vi "gui for machine parameters.vi"() -> ()   [LabVIEW 2022 SP3]
uses:
  <vilib>/picture/picture.llb/Draw True-Color Pixmap.vi
  horizontal slide control.ctl
  <vilib>/picture/picture.llb/imagedata.ctl
panel:
  in  "stop 3":bool
  in  "dimension size":i32
  in  "Tank 3":dbl(slide) scale=0.0..100.0
  in  "Tank 2":dbl(slide) scale=0.0..100.0
  in  "Table 3":string[][](table)
  in  "?":bool
  in  "?":bool
  in  "?":bool
  in  "?":bool
  in  "?":bool
  in  "?":bool
  in  "?":bool
  in  "?":bool
  out "image data 2":T1
  in  "path to PNG file 2":path=path "C:/Dhanush/Dhanush/Vehicle articulated (1).PNG"
  in  "Rotation Angle (degree) 2":dbl(knob) scale=-180.0..180.0
  in  "Scale 2":dbl(slide)=1.0 scale=0.1..10.0
  in  "stop 2":bool
  out "?":picture
  out "image data":T1
  in  "path to PNG file":path=path "C:/Dhanush/Dhanush/Vehicle articulated (1).PNG"
  in  "Rotation Angle (degree)":dbl(knob) scale=-180.0..180.0
  in  "Scale":dbl(slide)=1.0 scale=0.1..10.0
  in  "stop":bool
  out "?":picture
  out "?":T2 scale=0.0..100.0
  in  "Table 2":string[][](table)
  # "No of Cycles"
  # "Holding Time"
  # "Y axis Angle"
  # "Pressure"
  # "Automatic Mode Parameter Settings"
  # "Y axis"
  # "X axis"
  # "Cycle"
  # "Settings"
  # "%"
  # "Overall Progress Bar"
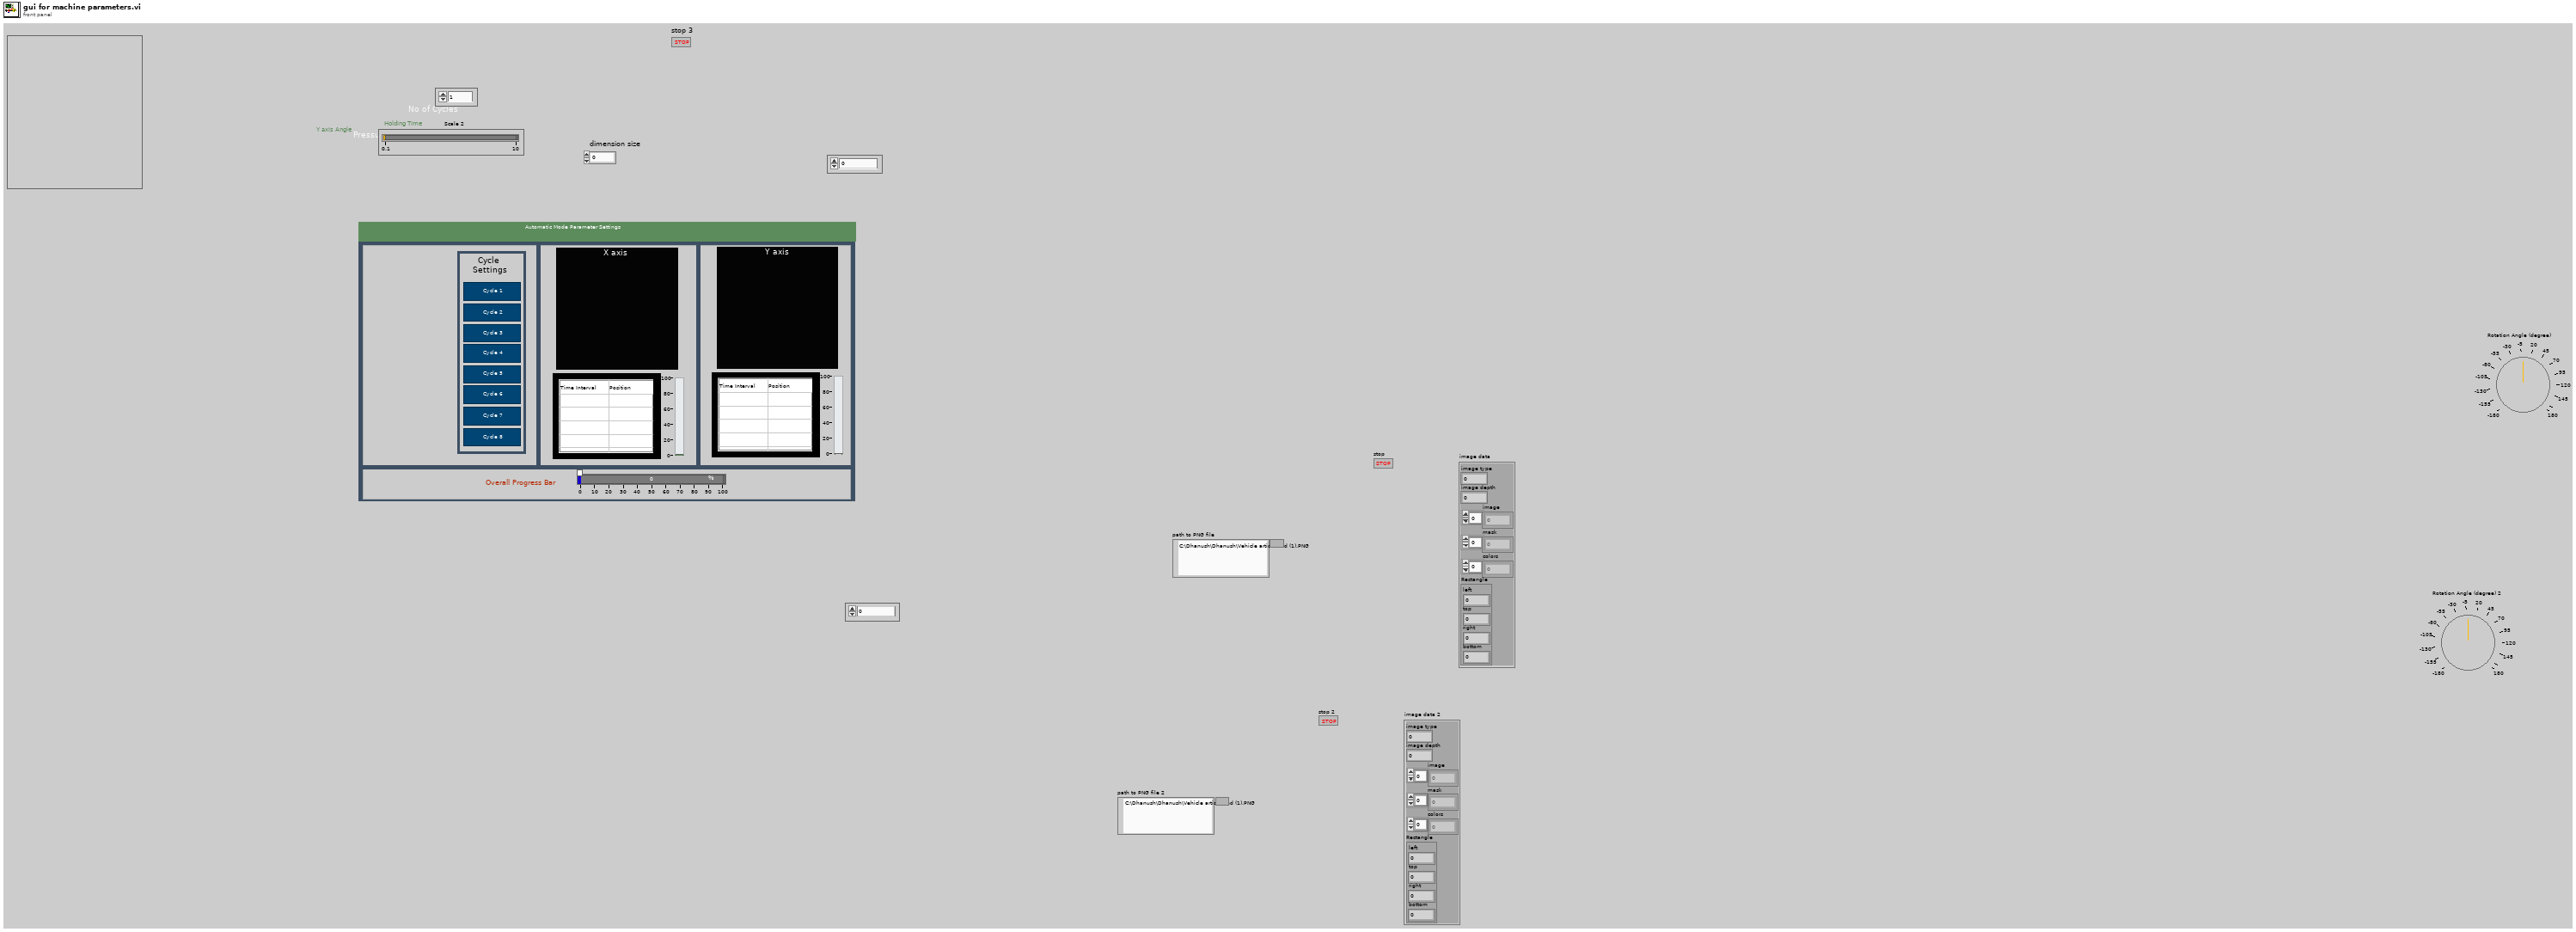
[diagram p1: front panel]
types:
  T1 = typedef "imagedata.ctl" = cluster{"image type":i32, "image depth":i32, "image":u8[], "mask":u8[], "colors":u32[], "Rectangle":cluster{"left":i16, "top":i16, "right":i16, "bottom":i16}}
  T2 = typedef "horizontal slide control.ctl" = dbl
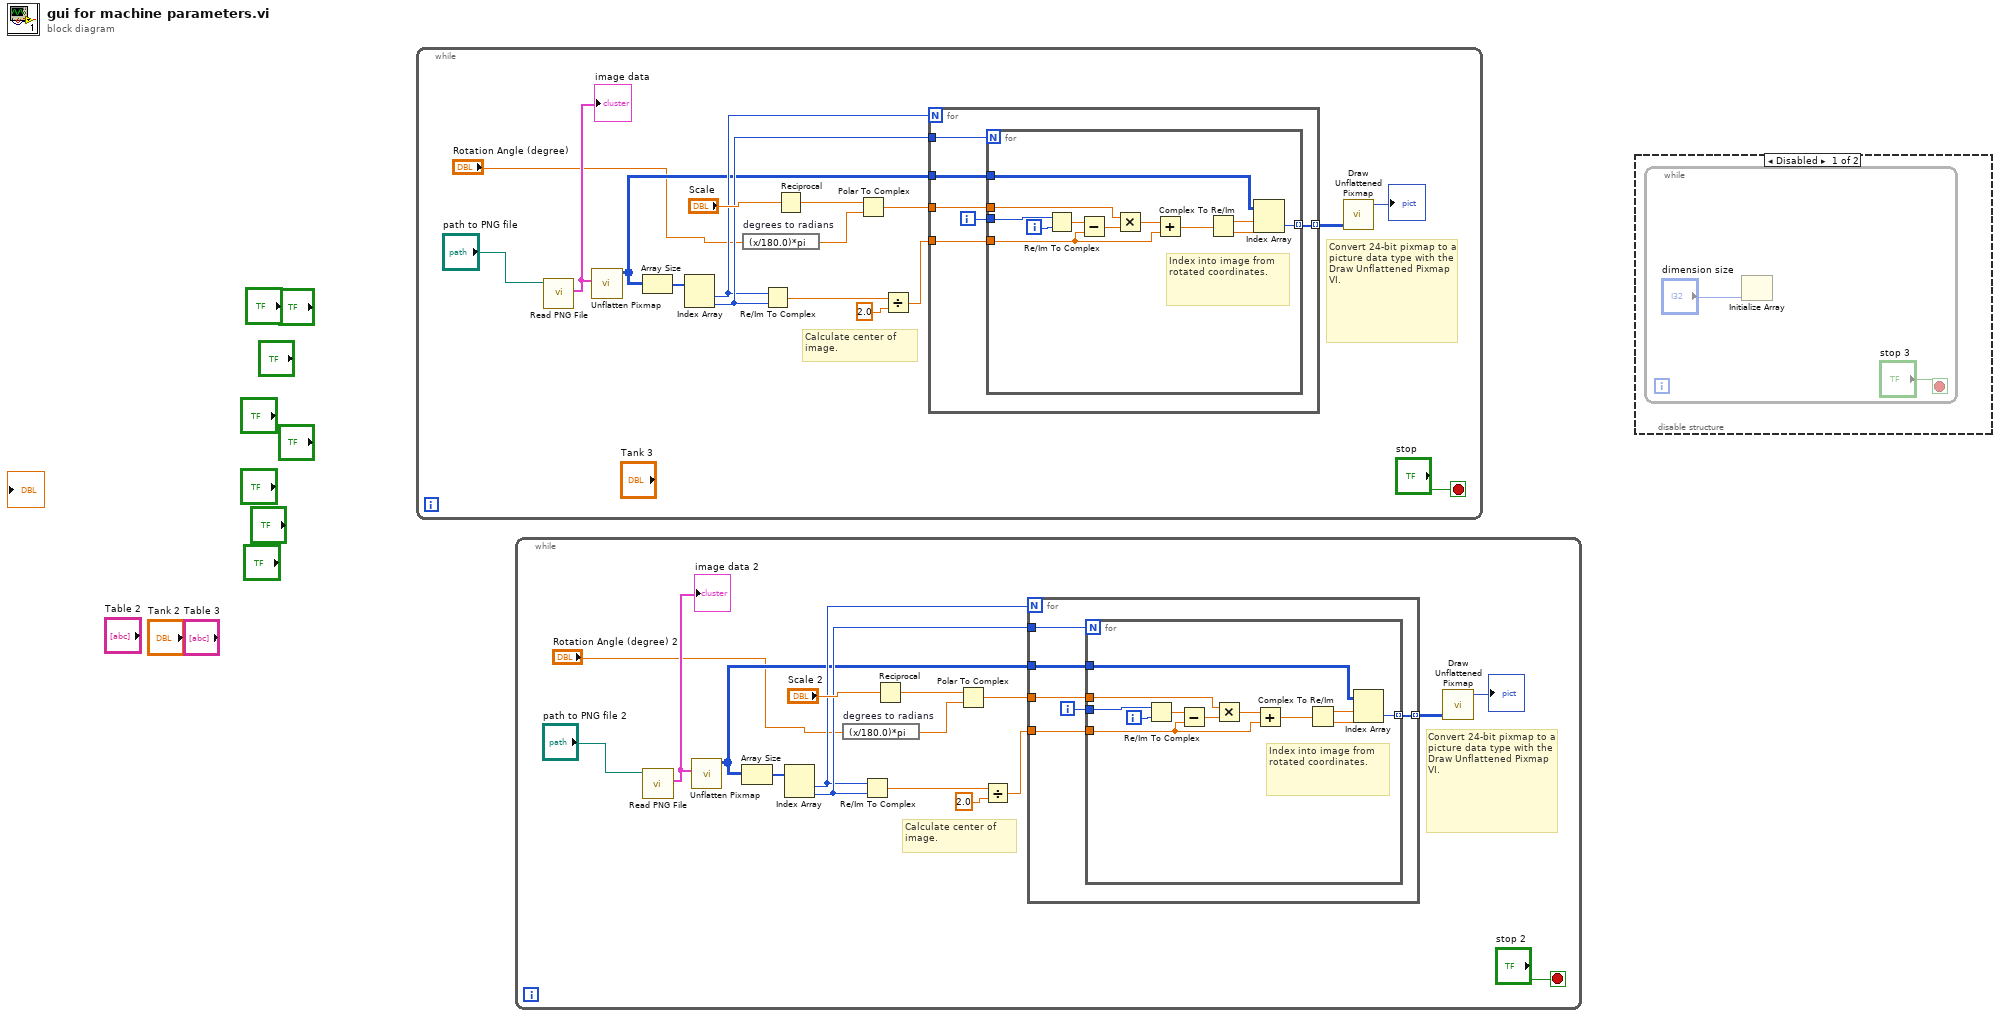
[diagram p0: block diagram]
diagram:
  n1 = while {
    stop <- "stop" stop-if-true
    # "Calculate center of image."
    # "Convert 24-bit pixmap to a picture data type with the Draw Unflattened Pixmap VI."
    n2 = call <vilib>:"Read PNG File.vi"("path to PNG file"="path to PNG file") -> ("image data"=w5:T1)  [unwired: 8 in, 2 out]
    "image data" <- w5
    n3 = call <vilib>:"Unflatten Pixmap.vi"("image data"=w5) -> ("24-bit pixmap"=w6:u32[][])  [unwired: 4 in, 6 out]
    n4 = Array Size(array=w6) -> (size(s)=w11:i32[])
    n5 = Index Array(array=w11) -> (element #1=w9:i32, element #2=w10:i32)  [unwired: 2 in]
    n6 = expression code="(x/180.0)*pi" "degrees to radians"("Rotation Angle (degree)") -> (w4:dbl)
    n7 = Re/Im To Complex(1:w10, 2:w9) -> (0:w12:cdb)
    n8 = Reciprocal(x="Scale") -> (1/x=w14:dbl)
    n9 = Polar To Complex(1:w4, 2:w14) -> (0:w13:cdb)
    n10 = Divide(x=w12, y=2.0) -> (x/y=w8:cdb)
    n11 = for {
      N: w9 -> [_]
      tunnel: w10 -> [w22]
      tunnel: w6 -> [w21]
      tunnel: [w20] -> w16 mode=indexing
      tunnel: w13 -> [w19]
      tunnel: w8 -> [w18]
      i -> [w23]
      n12 = for {
        N: w22 -> [_]
        tunnel: w23 -> [w32]
        tunnel: w21 -> [w35]
        tunnel: [w34] -> w20 mode=indexing
        tunnel: w19 -> [w25]
        tunnel: w18 -> [w24]
        i -> [w33]
        # "Index into image from rotated coordinates."
        n13 = Re/Im To Complex(1:w33, 2:w32) -> (0:w31:cdb)
        n14 = Subtract(x=w31, y=w24) -> (x-y=w30:cdb)
        n15 = Multiply(x=w25, y=w30) -> (x*y=w29:cdb)
        n16 = Add(x=w29, y=w24) -> (x+y=w28:cdb)
        n17 = Complex To Re/Im(x + iy=w28) -> (x=w27:dbl, y=w26:dbl)
        n18 = Index Array(array=w35, index (row)=w27, index (col)=w26) -> (element=w34:u32)
      }
    }
    n19 = call-poly <vilib>:"Draw Unflattened Pixmap.vi"("data (RGB format)"=w16) -> ("new picture"=→"?":picture)  [unwired: 8 in]
  }
  n20 = while {
    stop <- "stop 2" stop-if-true
    # "Calculate center of image."
    # "Convert 24-bit pixmap to a picture data type with the Draw Unflattened Pixmap VI."
    n21 = call <vilib>:"Read PNG File.vi"("path to PNG file"="path to PNG file 2") -> ("image data"=w40:T1)  [unwired: 8 in, 2 out]
    "image data 2" <- w40
    n22 = call <vilib>:"Unflatten Pixmap.vi"("image data"=w40) -> ("24-bit pixmap"=w41:u32[][])  [unwired: 4 in, 6 out]
    n23 = Array Size(array=w41) -> (size(s)=w46:i32[])
    n24 = Index Array(array=w46) -> (element #1=w44:i32, element #2=w45:i32)  [unwired: 2 in]
    n25 = expression code="(x/180.0)*pi" "degrees to radians"("Rotation Angle (degree) 2") -> (w39:dbl)
    n26 = Re/Im To Complex(1:w45, 2:w44) -> (0:w47:cdb)
    n27 = Reciprocal(x="Scale 2") -> (1/x=w49:dbl)
    n28 = Polar To Complex(1:w39, 2:w49) -> (0:w48:cdb)
    n29 = Divide(x=w47, y=2.0) -> (x/y=w43:cdb)
    n30 = for {
      N: w44 -> [_]
      tunnel: w45 -> [w57]
      tunnel: w41 -> [w56]
      tunnel: [w55] -> w51 mode=indexing
      tunnel: w48 -> [w54]
      tunnel: w43 -> [w53]
      i -> [w58]
      n31 = for {
        N: w57 -> [_]
        tunnel: w58 -> [w67]
        tunnel: w56 -> [w70]
        tunnel: [w69] -> w55 mode=indexing
        tunnel: w54 -> [w60]
        tunnel: w53 -> [w59]
        i -> [w68]
        # "Index into image from rotated coordinates."
        n32 = Re/Im To Complex(1:w68, 2:w67) -> (0:w66:cdb)
        n33 = Subtract(x=w66, y=w59) -> (x-y=w65:cdb)
        n34 = Multiply(x=w60, y=w65) -> (x*y=w64:cdb)
        n35 = Add(x=w64, y=w59) -> (x+y=w63:cdb)
        n36 = Complex To Re/Im(x + iy=w63) -> (x=w62:dbl, y=w61:dbl)
        n37 = Index Array(array=w70, index (row)=w62, index (col)=w61) -> (element=w69:u32)
      }
    }
    n38 = call-poly <vilib>:"Draw Unflattened Pixmap.vi"("data (RGB format)"=w51) -> ("new picture"=→"?":picture)  [unwired: 8 in]
  }
  n39 = disable-structure shown="Disabled" {
    frame Disabled {
      n40 = while {
        stop <- "stop 3" stop-if-true
        n41 = Initialize Array("dimension size") -> ()  [unwired: 1 in, 1 out]
      }
    }
    frame Enabled {
    }
  }
